vi "txt파일저장된 데이터 하나씩 분리.vi"(3 "파일(대화 상자 사용)":path) -> (0 "Lon":dbl format="%#.8g", 1 "Lat":dbl format="%#.8g")   [LabVIEW 2016]
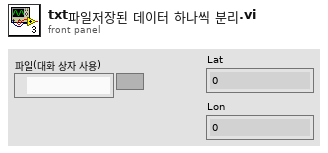
[diagram p1: front panel]
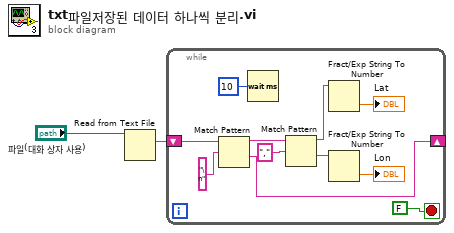
[diagram p0: block diagram]
diagram:
  n1 = Read from Text File(file (use dialog)="파일(대화 상자 사용)") -> (text=w2:string)  [unwired: 3 in, 3 out]
  n2 = while {
    shift-right: [w13] -> _
    shift-left: w2 -> [w12]
    stop <- FALSE stop-if-true
    n3 = Match Pattern(string=w12, regular expression="\n" ("정규식")) -> (before substring=w10:string, after substring=w13:string)  [unwired: 1 in, 2 out]
    n4 = Wait (ms)(milliseconds to wait=u32 10 ("대기 시간 (ms)")) -> ()  [unwired: 1 out]
    n5 = Match Pattern(string=w10, regular expression="," ("정규식")) -> (before substring=w8:string, after substring=w7:string)  [unwired: 1 in, 2 out]
    n6 = Fract/Exp String To Number(string=w8) -> (number=→"Lat":dbl)  [unwired: 3 in, 1 out]
    n7 = Fract/Exp String To Number(string=w7) -> (number=→"Lon":dbl)  [unwired: 3 in, 1 out]
  }
